vi "ROS send websock.vi"(8 "ConnectionIn":T2, 10 "Data in":T3, 11 "TELEMETRY type 2":T1) -> (0 "ConnectioOut":T2, 2 "rawJSONOut":string)   [LabVIEW 2015]
uses:
  Control  rossss.ctl
  <vilib>/MediaMongrels Ltd/WebSockets/WebSockets/WebSockets.lvlib
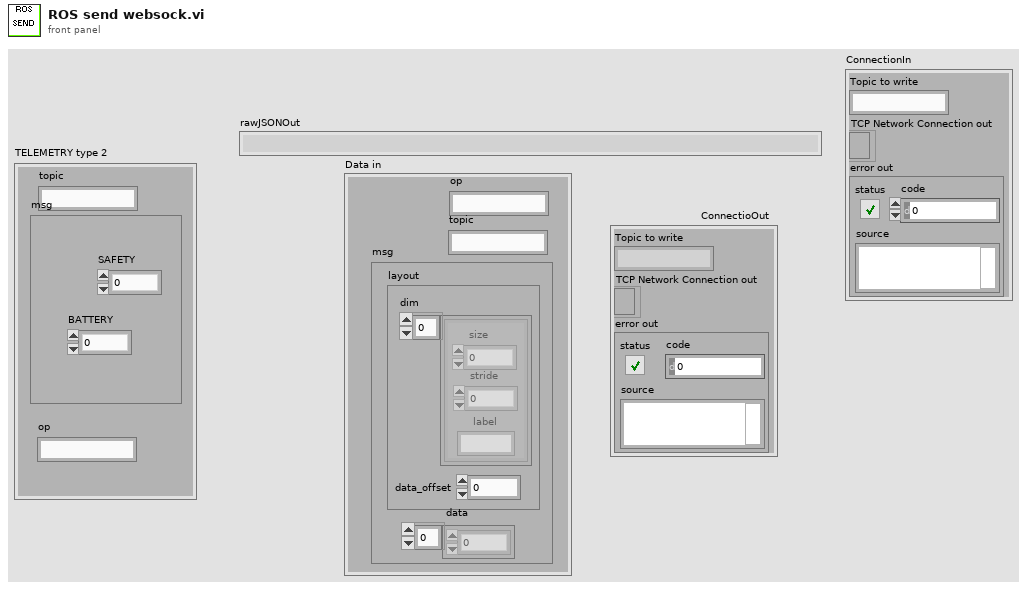
[diagram p1: front panel]
types:
  T1 = cluster{"topic":string, "msg":cluster{"SAFETY":i8, "BATTERY":i8}, "op":string}
  T2 = cluster{"Topic to write":string, "TCP Network Connection out":refnum<k5>, "error out":errorcluster}
  T3 = typedef "Control  rossss.ctl" = cluster{"op":string, "topic":string, "msg":cluster{"layout":cluster{"dim":cluster{"stride":i16, "size":i16, "label":string}[], "data_offset":dbl}, "data":i32[]}}
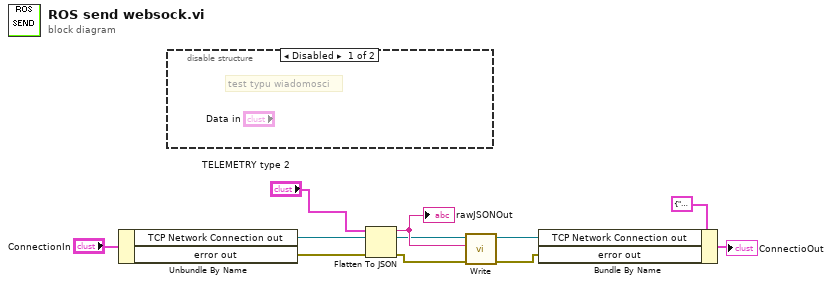
[diagram p0: block diagram]
diagram:
  n1 = Unbundle By Name("ConnectionIn") -> ("TCP Network Connection out"=w7:refnum<k5>, "error out"=w6:errorcluster)
  n2 = disable-structure shown="Disabled" {
    frame Disabled {
      # "test typu wiadomosci"
    }
    frame Enabled {
    }
  }
  n3 = Flatten To JSON(anything="TELEMETRY type 2", error in (no error)=w6) -> (JSON string=w9:string, 11:w10:errorcluster)  [unwired: 1 in]
  "rawJSONOut" <- w9
  n4 = call <vilib>:"Write.vi"("error in (no error)"=w10, "Data"=w9, "WebSocket Connection in"=w7) -> ("error out"=w3:errorcluster, "WebSocket Connection out"=w4:refnum<k5>)  [unwired: 7 in]
  n5 = Bundle By Name(cluster=T2 {"Topic to write"="", "TCP Network Connection out"=refnum, "error out"={"status"=FALSE, "code"=0, "source"=""}} ("output cluster 2"), "TCP Network Connection out"=w4, "error out"=w3) -> (→"ConnectioOut":T2)
